vi "External_Open Blockdiagram.vi"(8 "error in":errorcluster, 9 "Open":bool, 10 "VIs":string[](array[string]), 11 "Application in":refnum<vi>) -> (0 "error out":errorcluster)   [LabVIEW 2013]
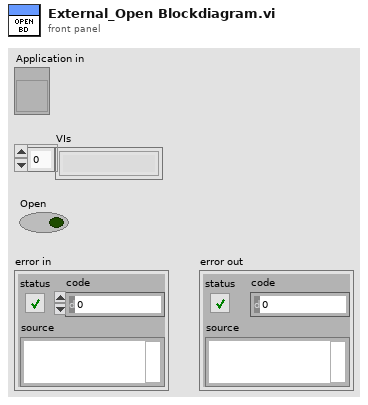
[diagram p1: front panel]
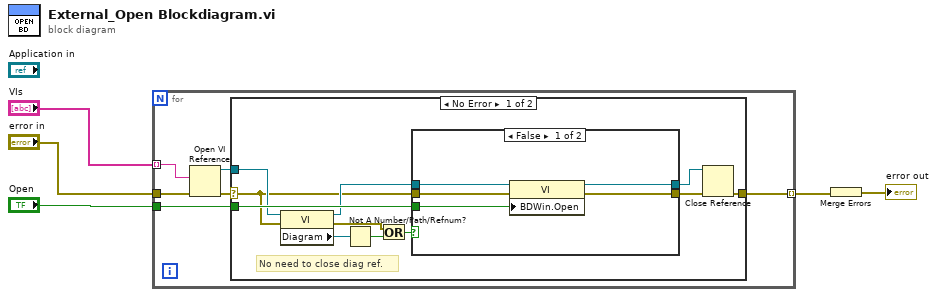
[diagram p0: block diagram]
diagram:
  n1 = for {
    tunnel: [w11] -> w2 mode=indexing
    tunnel: "error in" -> [w10]
    tunnel: "VIs" -> [w9] mode=indexing
    tunnel: "Open" -> [w8]
    n2 = Open VI Reference(vi path=w9, error in (no error)=w10) -> (vi reference=w7:refnum<vi>, error out=w6:errorcluster)  [unwired: 4 out]
    n3 = case shown="No Error" w6 {
      selector: w6 -> [w12 _]
      tunnel: [w22 _] -> w11
      tunnel: w8 -> [w19 _]
      tunnel: w7 -> [w18 _]
      frame No Error {
        # "No need to close diag ref."
        n4 = property class="VI"(reference=w18, error in=w12) -> (reference out=w17:refnum<vi>, error out=w14:errorcluster, "Diagram"=w16:refnum<vi>)
        n5 = Not A Number/Path/Refnum?(number/path/refnum=w16) -> (NaN/Path/Refnum?=w15:bool)
        n6 = Or(x=w14, y=w15) -> (x .or. y?=w13:bool)
        n7 = case shown="False" w13 {
          tunnel: [w27 w29] -> w21
          tunnel: [w26 w28] -> w20
          tunnel: w19 -> [w25 _]
          tunnel: w12 -> [w24 w28]
          tunnel: w17 -> [w23 w29]
          frame False {
            n8 = property class="VI"(reference=w23, error in=w24, "BDWin.Open"=w25) -> (reference out=w27:refnum<vi>, error out=w26:errorcluster)
          }
          frame True {
            # "VI saved without block diagram or is pwd protected."
          }
        }
        n9 = Close Reference(reference=w21, error in (no error)=w20) -> (error out=w22:errorcluster)
      }
      frame Error {
        # "This VI is no longer in the memory"
      }
    }
  }
  n10 = Merge Errors(w2) -> (→"error out":errorcluster)
